vi "Epoxy_InitializeBools.vi"(8 "error in (no error)":errorcluster, 11 "Data Cluster":T1) -> (0 "error out":errorcluster)   [LabVIEW 2020]
uses:
  controls/Valves Radio.ctl
  controls/Epoxy_CompEnable.ctl
  controls/UI Data.ctl
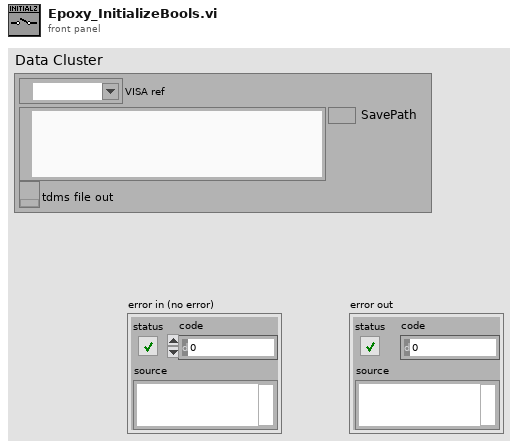
[diagram p1: front panel]
types:
  T1 = typedef "UI Data.ctl" = cluster{"VISA ref":refnum<visa-resource-name>, "SavePath":path, "tdms file out":refnum<k34>}
  T2 = typedef "Epoxy_CompEnable.ctl" = bool
  T3 = typedef "Valves Radio.ctl" = enum32{"A", "B"}
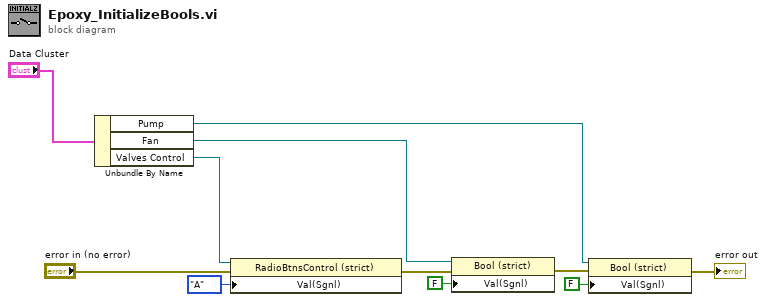
[diagram p0: block diagram]
diagram:
  n1 = Unbundle By Name("Data Cluster") -> ("Pump"=w2:refnum<vi>, "Fan"=w6:refnum<vi>, "Valves Control"=w10:refnum<vi>)
  n2 = property class="RadioBtnsControl (strict)"(reference=w10, error in="error in (no error)", "Val(Sgnl)"=Valves_Radio."A" ("Value (Signaling)")) -> (error out=w7:errorcluster)  [unwired: 1 out]
  n3 = property class="Bool (strict)"(reference=w6, error in=w7, "Val(Sgnl)"=T2 FALSE ("Value (Signaling)")) -> (error out=w1:errorcluster)  [unwired: 1 out]
  n4 = property class="Bool (strict)"(reference=w2, error in=w1, "Val(Sgnl)"=T2 FALSE ("Value (Signaling)")) -> (error out=→"error out":errorcluster)  [unwired: 1 out]
